vi "XNET Reflective Memory Main Page.vi"(8 "error in (no error)":errorcluster, 11 "Node Ptr":T1 format="%.0x") -> (0 "error out":errorcluster)   [LabVIEW 2010, in "XNET Reflective Memory Custom Device.lvlib"]
uses:
  XNET Reflective Memory Custom Device.lvlib
  <vilib>/NI VeriStand/Custom Device API/Custom Device Item Ref.ctl
  Global.vi
  <vilib>/NI VeriStand/Custom Device API/Get Item Property (Boolean).vi
  <vilib>/NI VeriStand/Custom Device API/Get Item Property (U32).vi
  <vilib>/NI VeriStand/Custom Device API/Get Item Property (String).vi
  <vilib>/NI VeriStand/Custom Device API/Set Item Property (String).vi
  <vilib>/NI VeriStand/Custom Device API/Set Item Property (U32).vi
  <vilib>/NI VeriStand/Custom Device API/Set Item Property (Boolean).vi
  <vilib>/NI Veristand/Custom Device API/Custom Device API.lvlib
panel:
  in  "Start Trigger":bool
  in  "Cluster":string
  in  "Database":string
  in  "Cold Start?":bool
  in  "Key Slot Identifier":u32
  in  "FlexRay Interface":string
  in  "Header":cluster{"Section Name":string}={"Section Name"="Custom Device Item Settings"}
  in  "Description":string
  in  "Name":string
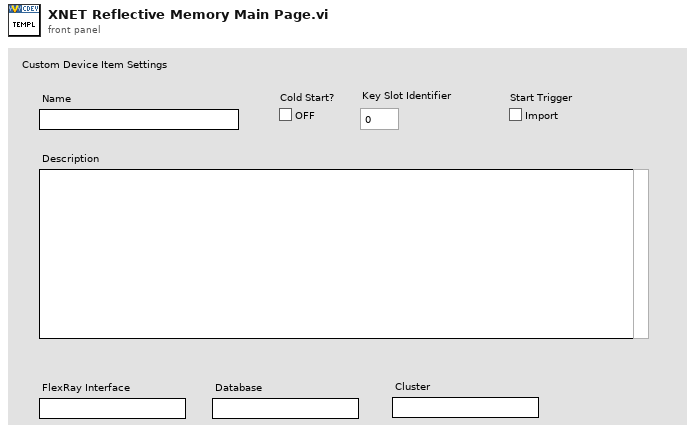
[diagram p1: front panel]
types:
  T1 = typedef "Custom Device API.lvlib/Custom Device Item Ref.ctl" = u64
  T2 = enum8{"Enabled", "Disabled", "Disabled and Grayed Out"}
  T3 = typedef "Custom Device API.lvlib/Custom Device Item Info.ctl" = cluster{"Name":string, "Is Channel":bool, "GUID":string}
  T4 = typedef "Custom Device API.lvlib/Custom Device Commands.ctl" = enum16{"Default", "Item renamed", "Shutdown", "Dynamic button pressed"}
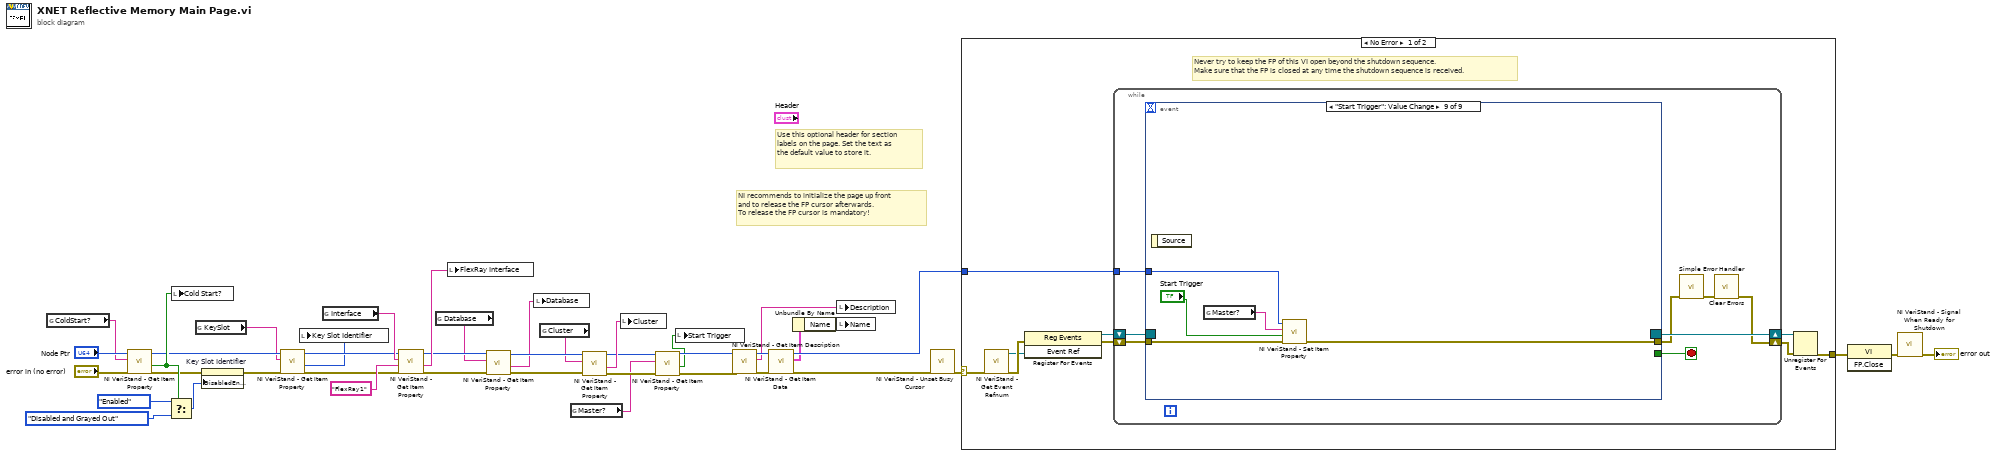
[diagram p0: block diagram]
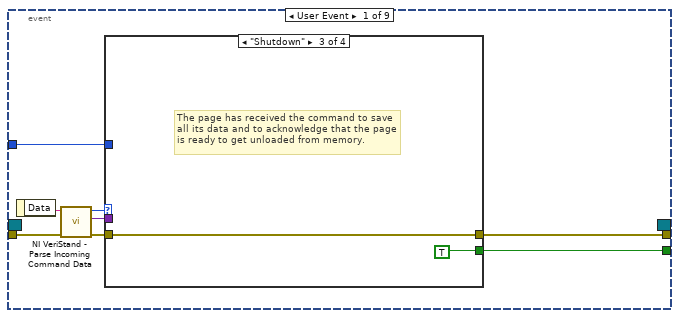
[diagram p2: hidden frame]
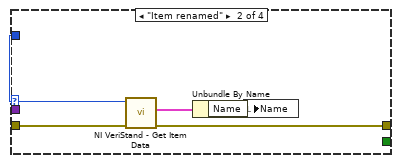
[diagram p4: hidden frame]
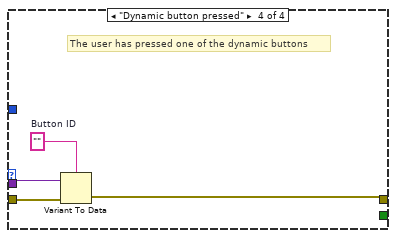
[diagram p5: hidden frame]
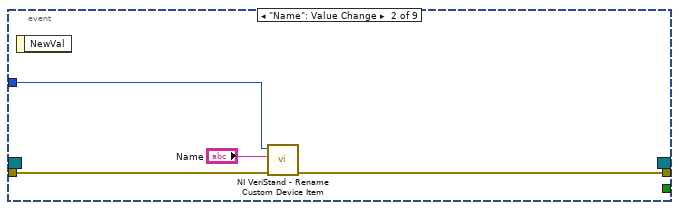
[diagram p6: hidden frame]
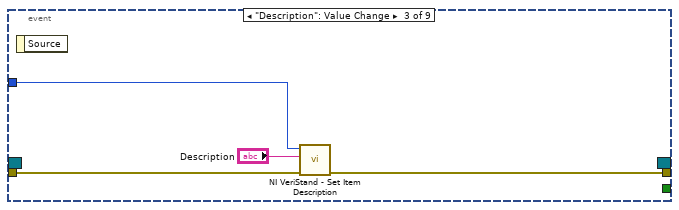
[diagram p7: hidden frame]
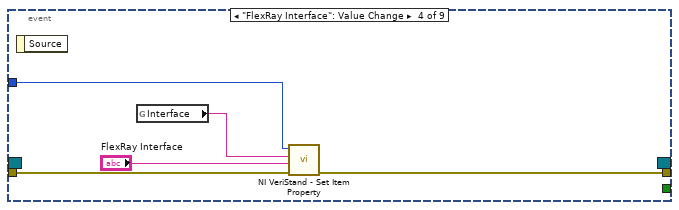
[diagram p8: hidden frame]
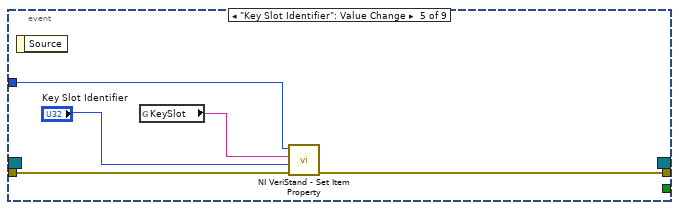
[diagram p9: hidden frame]
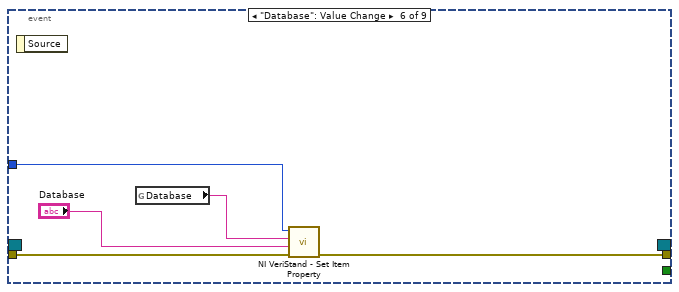
[diagram p10: hidden frame]
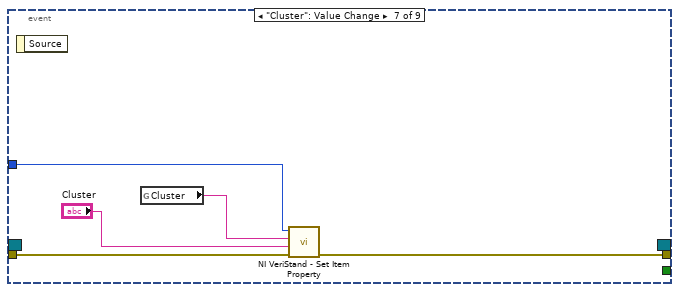
[diagram p11: hidden frame]
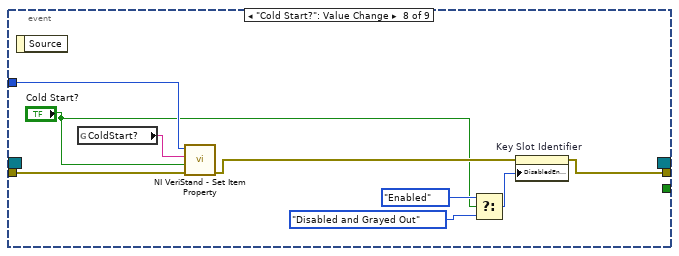
[diagram p12: hidden frame]
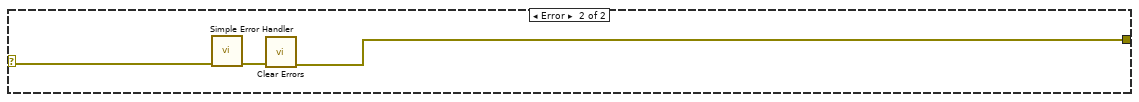
[diagram p13: hidden frame]
diagram:
  # "Use this optional header for section labels on the page. Set the text as the default value to store it."
  # "NI recommends to initialize the page up front\nand to release the FP cursor afterwards.\nTo release the FP cursor is mandatory!"
  n1 = global read "Global.vi" "ColdStart?"() -> (w26:string)
  n2 = call-poly <vilib>:"NI VeriStand - Get Item Property.vi"("error in (no error)"="error in (no error)", "Property Name"=w26, "Item Ref in"="Node Ptr") -> ("error out"=w24:errorcluster, "Value"=w25:bool, "Item Ref out"=w19:T1)  [unwired: 5 in, 1 out]
  n3 = Select(t=T2."Enabled" ("Disabled"), s=w25, f=T2."Disabled and Grayed Out" ("Disabled")) -> (s? t:f=w23:T2)
  n4 = local write "Cold Start?"(w25) -> ()
  n5 = global read "Global.vi" "KeySlot"() -> (w18:string)
  n6 = property on="Key Slot Identifier" class="DigNum (strict)"(error in=w24, "DisabledEnum"=w23) -> (error out=w20:errorcluster)  [unwired: 1 in, 1 out]
  n7 = call-poly <vilib>:"NI VeriStand - Get Item Property.vi"("error in (no error)"=w20, "Property Name"=w18, "Item Ref in"=w19) -> ("error out"=w17:errorcluster, "Value"=w15:u32, "Item Ref out"=w16:T1)  [unwired: 5 in, 1 out]
  n8 = local write "Key Slot Identifier"(w15) -> ()
  n9 = global read "Global.vi" "Interface"() -> (w31:string)
  n10 = call-poly <vilib>:"NI VeriStand - Get Item Property.vi"("error in (no error)"=w17, "Default Value"="FlexRay1", "Property Name"=w31, "Item Ref in"=w16) -> ("error out"=w14:errorcluster, "Value"=w29:string, "Item Ref out"=w13:T1)  [unwired: 4 in, 1 out]
  n11 = global read "Global.vi" "Database"() -> (w10:string)
  n12 = local write "FlexRay Interface"(w29) -> ()
  n13 = call-poly <vilib>:"NI VeriStand - Get Item Property.vi"("error in (no error)"=w14, "Property Name"=w10, "Item Ref in"=w13) -> ("error out"=w11:errorcluster, "Value"=w9:string, "Item Ref out"=w12:T1)  [unwired: 5 in, 1 out]
  n14 = local write "Database"(w9) -> ()
  n15 = global read "Global.vi" "Cluster"() -> (w8:string)
  n16 = global read "Global.vi" "Master?"() -> (w4:string)
  n17 = call-poly <vilib>:"NI VeriStand - Get Item Property.vi"("error in (no error)"=w11, "Property Name"=w8, "Item Ref in"=w12) -> ("error out"=w6:errorcluster, "Value"=w7:string, "Item Ref out"=w5:T1)  [unwired: 5 in, 1 out]
  n18 = local write "Cluster"(w7) -> ()
  n19 = call-poly <vilib>:"NI VeriStand - Get Item Property.vi"("error in (no error)"=w6, "Property Name"=w4, "Item Ref in"=w5) -> ("error out"=w3:errorcluster, "Value"=w1:bool, "Item Ref out"=w2:T1)  [unwired: 5 in, 1 out]
  n20 = local write "Start Trigger"(w1) -> ()
  n21 = call <vilib>:"NI VeriStand - Get Item Description.vi"("error in (no error)"=w3, "Item Ref in"=w2) -> ("error out"=w34:errorcluster, "Description"=w35:string, "Item Ref out"=w36:T1)  [unwired: 7 out]
  n22 = call <vilib>:"NI VeriStand - Get Item Data.vi"("error in (no error)"=w34, "Item Ref in"=w36) -> ("error out"=w39:errorcluster, "Item Info"=w33:T3, "Item Ref out"=w37:T1)  [unwired: 7 out]
  n23 = Unbundle By Name(w33) -> ("Name"=w32:string)
  n24 = local write "Description"(w35) -> ()
  n25 = local write "Name"(w32) -> ()
  n26 = call <vilib>:"NI VeriStand - Unset Busy Cursor.vi"("error in (no error)"=w39) -> ("error out"=w38:errorcluster)  [unwired: 10 out]
  n27 = case shown="No Error" w38 {
    selector: w38 -> [w43 w124]
    tunnel: [w48 w122] -> w42
    tunnel: w37 -> [w44 _]
    frame No Error {
      # "Never try to keep the FP of this VI open beyond the shutdown sequence.\nMake sure that the FP is closed at any time the shutdown sequence is received."
      n28 = call <vilib>:"NI VeriStand - Get Event Refnum.vi"("error in (no error)"=w43) -> ("error out"=w51:errorcluster, "Event Ref"=w47:refnum<user-event>)  [unwired: 9 out]
      n29 = register-events(error in=w51, w47) -> (reference out=w45:refnum<event-registration>, error out=w46:errorcluster)  [unwired: 1 in]
      n30 = while {
        tunnel: w44 -> [w55]
        shift-right: [w52] -> w49
        shift-left: w46 -> [w58]
        shift-right: [w59] -> w50
        shift-left: w45 -> [w57]
        stop <- w56 stop-if-true
        n31 = event shown="[8] \"Start Trigger\": Value Change" {
          selector: w57 -> [_ _ _ _ _ _ _ _ _]
          dyn-events: [_ _ _ _ _ _ _ _ _] -> w59
          timeout: _ -> [_ _ _ _ _ _ _ _ _]
          tunnel: w58 -> [w67 w83 w86 w92 w97 w102 w107 w116 w121]
          tunnel: [w63 _ _ _ _ _ _ _ _] -> w56
          tunnel: [w62 w82 w85 w91 w96 w101 w106 w109 w117] -> w54
          tunnel: w55 -> [w61 w81 w87 w90 w95 w100 w105 w115 w120]
          event User Event {
            n32 = event-data() -> ("Data"=w66:string)  [unwired: 1 out]
            n33 = call <vilib>:"NI VeriStand - Parse Incoming Command Data.vi"("error in (no error)"=w67, "Data"=w66) -> ("error out"=w65:errorcluster, "Data"=w60:variant, "Action"=w64:T4)  [unwired: 7 out]
            n34 = case shown="\"Shutdown\"" w64 {
              tunnel: w65 -> [w68 w73 w74 w79]
              tunnel: [_ _ TRUE _] -> w63
              tunnel: [w68 w70 w74 w76] -> w62
              tunnel: w61 -> [_ w72 _ _]
              tunnel: w60 -> [_ _ _ w78]
              frame "Default", Default {
              }
              frame "Item renamed" {
                n35 = call <vilib>:"NI VeriStand - Get Item Data.vi"("error in (no error)"=w73, "Item Ref in"=w72) -> ("error out"=w70:errorcluster, "Item Info"=w71:T3)  [unwired: 8 out]
                n36 = Unbundle By Name(w71) -> ("Name"=w69:string)
                n37 = local write "Name"(w69) -> ()
              }
              frame "Shutdown" {
                # "The page has received the command to save all its data and to acknowledge that the page is ready to get unloaded from memory."
              }
              frame "Dynamic button pressed" {
                w77 = ""  # Button ID
                # "The user has pressed one of the dynamic buttons"
                n38 = Variant To Data(error in=w79, Variant=w78, type=w77) -> (error out=w76:errorcluster)  [unwired: 1 out]
              }
            }
          }
          event "Name": Value Change {
            n39 = event-data() -> ()  [unwired: 2 out]
            n40 = call <vilib>:"NI VeriStand - Rename Custom Device Item.vi"("error in (no error)"=w83, "New Name"="Name", "Item Ref in"=w81) -> ("error out"=w82:errorcluster)  [unwired: 8 out]
          }
          event "Description": Value Change {
            n41 = event-data() -> ()  [unwired: 2 out]
            n42 = call <vilib>:"NI VeriStand - Set Item Description.vi"("error in (no error)"=w86, "Description"="Description", "Item Ref in"=w87) -> ("error out"=w85:errorcluster)  [unwired: 8 out]
          }
          event "FlexRay Interface": Value Change {
            n43 = event-data() -> ()  [unwired: 2 out]
            n44 = global read "Global.vi" "Interface"() -> (w89:string)
            n45 = call-poly <vilib>:"NI VeriStand - Set Item Property.vi"("error in (no error)"=w92, "Value"="FlexRay Interface", "Property Name"=w89, "Item Ref in"=w90) -> ("error out"=w91:errorcluster)  [unwired: 5 in, 2 out]
          }
          event "Key Slot Identifier": Value Change {
            n46 = event-data() -> ()  [unwired: 2 out]
            n47 = global read "Global.vi" "KeySlot"() -> (w94:string)
            n48 = call-poly <vilib>:"NI VeriStand - Set Item Property.vi"("error in (no error)"=w97, "Value"="Key Slot Identifier", "Property Name"=w94, "Item Ref in"=w95) -> ("error out"=w96:errorcluster)  [unwired: 5 in, 2 out]
          }
          event "Database": Value Change {
            n49 = event-data() -> ()  [unwired: 2 out]
            n50 = global read "Global.vi" "Database"() -> (w99:string)
            n51 = call-poly <vilib>:"NI VeriStand - Set Item Property.vi"("error in (no error)"=w102, "Value"="Database", "Property Name"=w99, "Item Ref in"=w100) -> ("error out"=w101:errorcluster)  [unwired: 5 in, 2 out]
          }
          event "Cluster": Value Change {
            n52 = event-data() -> ()  [unwired: 2 out]
            n53 = global read "Global.vi" "Cluster"() -> (w104:string)
            n54 = call-poly <vilib>:"NI VeriStand - Set Item Property.vi"("error in (no error)"=w107, "Value"="Cluster", "Property Name"=w104, "Item Ref in"=w105) -> ("error out"=w106:errorcluster)  [unwired: 5 in, 2 out]
          }
          event "Cold Start?": Value Change {
            n55 = event-data() -> ()  [unwired: 2 out]
            n56 = global read "Global.vi" "ColdStart?"() -> (w114:string)
            n57 = call-poly <vilib>:"NI VeriStand - Set Item Property.vi"("error in (no error)"=w116, "Value"="Cold Start?", "Property Name"=w114, "Item Ref in"=w115) -> ("error out"=w110:errorcluster)  [unwired: 5 in, 2 out]
            n58 = Select(t=T2."Enabled" ("Disabled"), s="Cold Start?", f=T2."Disabled and Grayed Out" ("Disabled")) -> (s? t:f=w111:T2)
            n59 = property on="Key Slot Identifier" class="DigNum (strict)"(error in=w110, "DisabledEnum"=w111) -> (error out=w109:errorcluster)  [unwired: 1 in, 1 out]
          }
          event "Start Trigger": Value Change {
            n60 = event-data() -> ()  [unwired: 2 out]
            n61 = global read "Global.vi" "Master?"() -> (w119:string)
            n62 = call-poly <vilib>:"NI VeriStand - Set Item Property.vi"("error in (no error)"=w121, "Value"="Start Trigger", "Property Name"=w119, "Item Ref in"=w120) -> ("error out"=w117:errorcluster)  [unwired: 5 in, 2 out]
          }
        }
        n63 = call <vilib>:"Simple Error Handler.vi"("error in (no error)"=w54) -> ("error out"=w53:errorcluster)  [unwired: 1 in, 7 out]
        n64 = call <vilib>:"Clear Errors.vi"("error in (no error)"=w53) -> ("error out"=w52:errorcluster)  [unwired: 6 out]
      }
      n65 = Unregister For Events(event registration refnum=w50, error in=w49) -> (error out=w48:errorcluster)
    }
    frame Error {
      n66 = call <vilib>:"Simple Error Handler.vi"("error in (no error)"=w124) -> ("error out"=w123:errorcluster)  [unwired: 1 in, 7 out]
      n67 = call <vilib>:"Clear Errors.vi"("error in (no error)"=w123) -> ("error out"=w122:errorcluster)  [unwired: 6 out]
    }
  }
  n68 = invoke class="VI" method="FP.Close"(error in=w42) -> (error out=w41:errorcluster)  [unwired: 2 in, 2 out]
  n69 = call <vilib>:"NI VeriStand - Signal When Ready for Shutdown.vi"("error in (no error)"=w41) -> ("error out"=→"error out":errorcluster)  [unwired: 10 out]
